vi "GetEnabledChains.vi"(1 "ChainMask":u8 format="0x%02x") -> (0 "Array":u8[](array[numeric]))   [LabVIEW 2023, in "ArduinoSerialBling.lvlib"]
uses:
  ArduinoSerialBling.lvlib
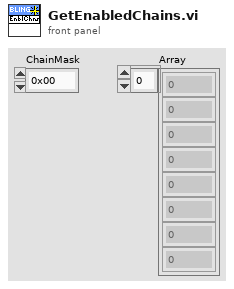
[diagram p1: front panel]
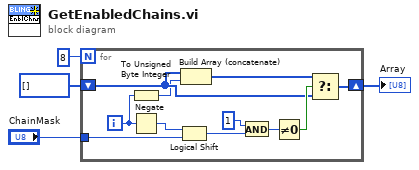
[diagram p0: block diagram]
diagram:
  n1 = for {
    N: 8 -> [_]
    shift-right: [w10] -> w4
    shift-left: u8[] [] -> [w11]
    tunnel: "ChainMask" -> [w8]
    i -> [w5]
    n2 = To Unsigned Byte Integer(number=w5) -> (unsigned 8bit integer=w7:u8)
    n3 = Negate(x=w5) -> (-x=w6:i32)
    n4 = Logical Shift(y=w6, x=w8) -> (x << y=w9:u8)
    n5 = Build Array (concatenate)(w11, w7) -> (w12:u8[])
    n6 = And(x=u8 1, y=w9) -> (x .and. y?=w14:u8)
    n7 = Not Equal To 0?(x=w14) -> (x != 0?=w13:bool)
    n8 = Select(t=w12, s=w13, f=w11) -> (s? t:f=w10:u8[])
  }
  "Array" <- w4
